vi "Configure Measurement1.vi"(6 "Manual Range (1)":dbl=1.0, 7 "Absolute Resolution (1E-6)":dbl=1e-06, 8 "error in (no error)":errorcluster, 9 "Auto Range (T: Enable)":bool=TRUE, 10 "Measurement Function (10: Voltage DC)":i32(ring)=10 items=["Continuity", "Current AC", "Current DC", "Diode", "Frequency", "Resistance 4-wire", "Period", "Resistance 2-wire", "Temperature", "Voltage AC", "Voltage DC", "Voltage DC Ratio"], 11 "VISA resource name":refnum<visa-resource-name>) -> (0 "error out":errorcluster, 3 "VISA resource name out":refnum<visa-resource-name>)   [LabVIEW 2015, in "Agilent 3446X Series1.lvlib"]
doc: "Configures the measurement type, resolution, and range on the instrument."
uses:
  Agilent 3446X Series1.lvlib
panel:
  out "Error Message":string
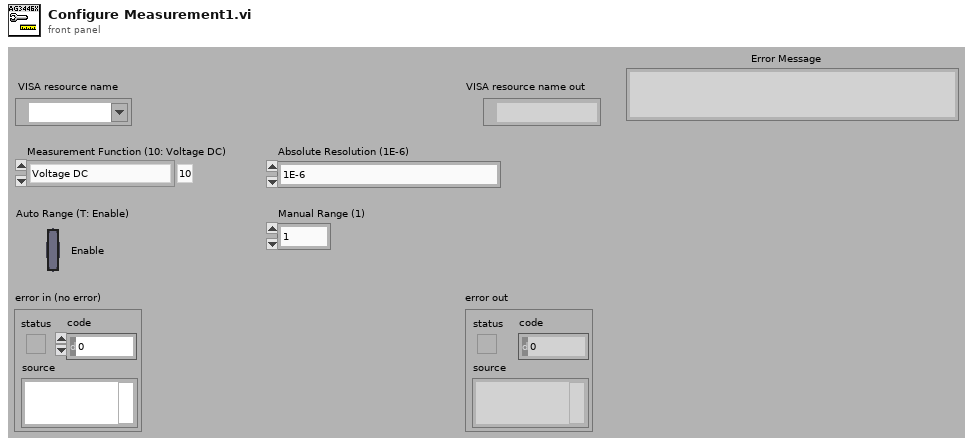
[diagram p1: front panel]
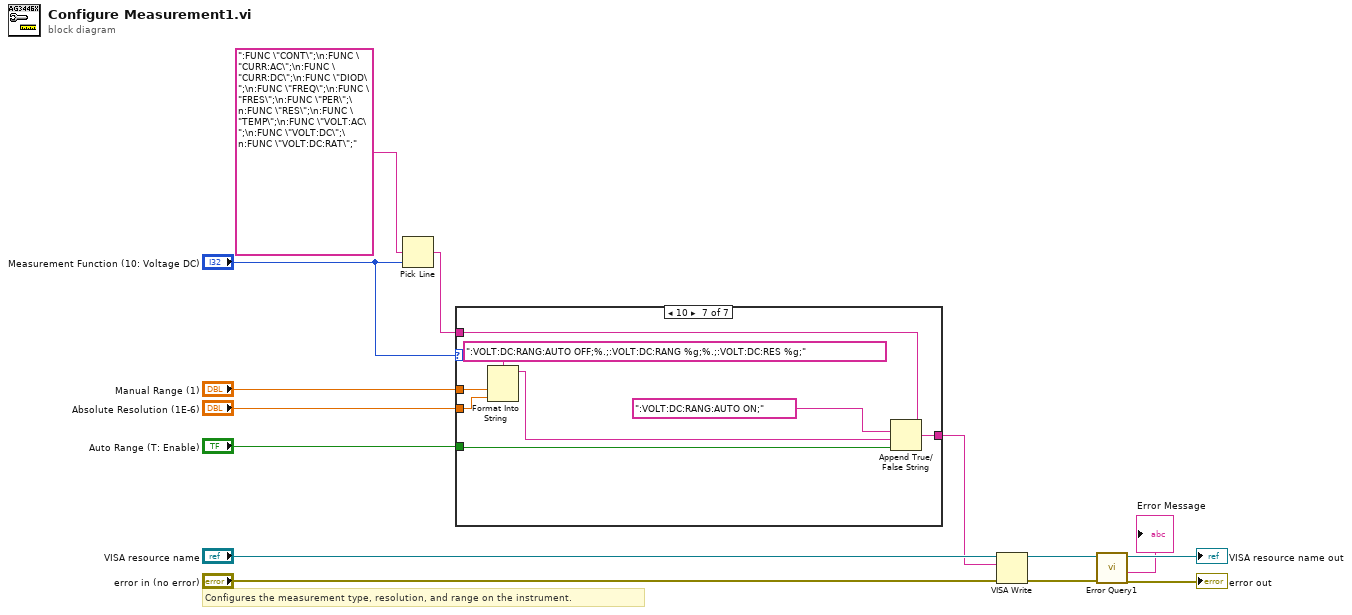
[diagram p0: block diagram]
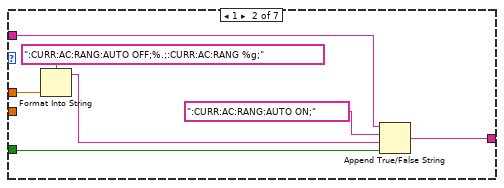
[diagram p3: hidden frame]
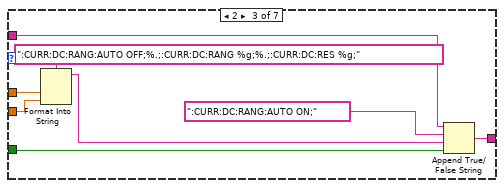
[diagram p4: hidden frame]
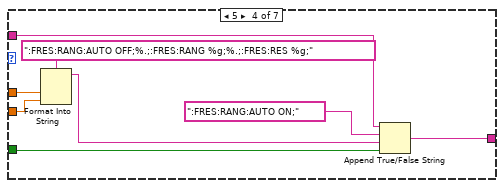
[diagram p5: hidden frame]
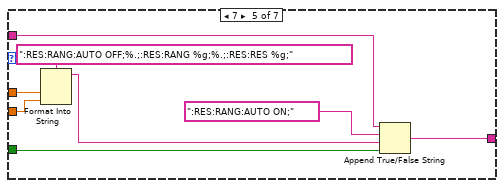
[diagram p6: hidden frame]
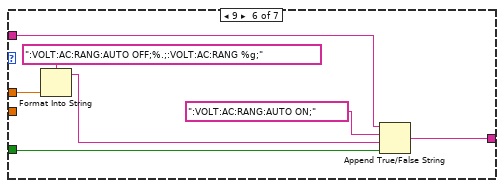
[diagram p7: hidden frame]
diagram:
  # "Configures the measurement type, resolution, and range on the instrument."
  n1 = Pick Line(multi-line string=":FUNC \"CONT\";\n:FUNC \"CURR:AC\";\n:FUNC \"CURR:DC\";\n:FUNC \"DIOD\";\n:FUNC \"FREQ\";\n:FUNC \"FRES\";\n:FUNC \"PER\";\n:FUNC \"RES\";\n:FUNC \"TEMP\";\n:FUNC \"VOLT:AC\";\n:FUNC \"VOLT:DC\";\n:FUNC \"VOLT:DC:RAT\";", line index="Measurement Function (10: Voltage DC)") -> (output string=w4:string)  [unwired: 1 out]
  n2 = case shown="10" "Measurement Function (10: Voltage DC)" {
    tunnel: "Manual Range (1)" -> [_ w21 w29 w37 w45 w52 w60]
    tunnel: "Auto Range (T: Enable)" -> [_ w18 w26 w34 w42 w49 w56]
    tunnel: w4 -> [w15 w17 w25 w33 w41 w48 w57]
    tunnel: [w15 w16 w23 w31 w40 w47 w54] -> w2
    tunnel: "Absolute Resolution (1E-6)" -> [_ _ w24 w32 w39 _ w55]
    frame 0, 3, 4, 6, 8, 11, Default {
    }
    frame 1 {
      n3 = Format Into String(format string=":CURR:AC:RANG:AUTO OFF;%.;:CURR:AC:RANG %g;", w21) -> (resulting string=w19:string)  [unwired: 2 in, 1 out]
      n4 = Append True/False String(1:w18, 2:w19, 3:":CURR:AC:RANG:AUTO ON;", 4:w17) -> (0:w16:string)
    }
    frame 2 {
      n5 = Format Into String(format string=":CURR:DC:RANG:AUTO OFF;%.;:CURR:DC:RANG %g;%.;:CURR:DC:RES %g;", w29, w24) -> (resulting string=w27:string)  [unwired: 2 in, 1 out]
      n6 = Append True/False String(1:w26, 2:w27, 3:":CURR:DC:RANG:AUTO ON;", 4:w25) -> (0:w23:string)
    }
    frame 5 {
      n7 = Format Into String(format string=":FRES:RANG:AUTO OFF;%.;:FRES:RANG %g;%.;:FRES:RES %g;", w37, w32) -> (resulting string=w35:string)  [unwired: 2 in, 1 out]
      n8 = Append True/False String(1:w34, 2:w35, 3:":FRES:RANG:AUTO ON;", 4:w33) -> (0:w31:string)
    }
    frame 7 {
      n9 = Format Into String(format string=":RES:RANG:AUTO OFF;%.;:RES:RANG %g;%.;:RES:RES %g;", w45, w39) -> (resulting string=w43:string)  [unwired: 2 in, 1 out]
      n10 = Append True/False String(1:w42, 2:w43, 3:":RES:RANG:AUTO ON;", 4:w41) -> (0:w40:string)
    }
    frame 9 {
      n11 = Format Into String(format string=":VOLT:AC:RANG:AUTO OFF;%.;:VOLT:AC:RANG %g;", w52) -> (resulting string=w50:string)  [unwired: 2 in, 1 out]
      n12 = Append True/False String(1:w49, 2:w50, 3:":VOLT:AC:RANG:AUTO ON;", 4:w48) -> (0:w47:string)
    }
    frame 10 {
      n13 = Format Into String(format string=":VOLT:DC:RANG:AUTO OFF;%.;:VOLT:DC:RANG %g;%.;:VOLT:DC:RES %g;", w60, w55) -> (resulting string=w58:string)  [unwired: 2 in, 1 out]
      n14 = Append True/False String(1:w56, 2:w58, 3:":VOLT:DC:RANG:AUTO ON;", 4:w57) -> (0:w54:string)
    }
  }
  n15 = VISA Write(VISA resource name="VISA resource name", write buffer=w2, error in (no error)="error in (no error)") -> (VISA resource name out=w11:refnum<visa-resource-name>, error out=w10:errorcluster)  [unwired: 1 out]
  n16 = call "Error Query1.vi"("error in (no error)"=w10, "VISA resource name"=w11) -> ("error out"=→"error out":errorcluster, "Error Message"=→"Error Message":string, "VISA resource name out"=→"VISA resource name out":refnum<visa-resource-name>)  [unwired: 7 out]
